vi "Write Frame (Binary).vi"(8 "error in (no error)":errorcluster, 9 "timeout (1000 ms)":i32=1000, 10 "Bytes":u8[](array[numeric]) format="%08b", 11 "Connection.WS":refnum<class "Connection.WS.lvclass">) -> (0 "error out":errorcluster, 3 "Connection.WS":refnum<class "Connection.WS.lvclass">)   [LabVIEW 2013, in "Connection.WS_GOSPL.lvlib" / "Connection.WS.lvclass"]
uses:
  Connection.WS.lvclass
  Websocket Frame Type -- ring.ctl
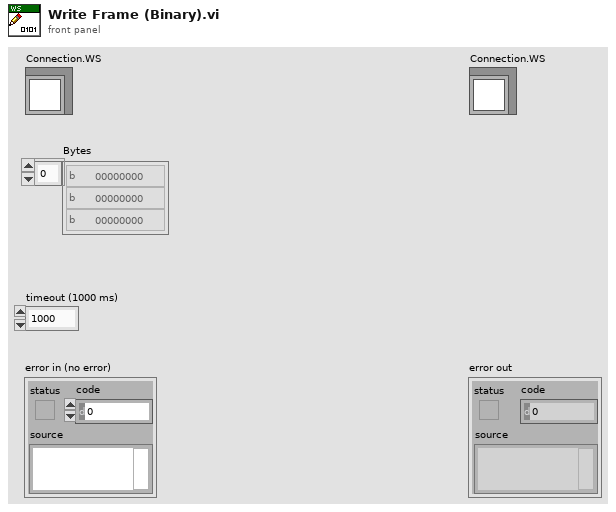
[diagram p1: front panel]
types:
  T1 = typedef "Connection.WS_GOSPL.lvlib/Connection.WS.lvclass/Websocket Frame Type -- ring.ctl" = u8
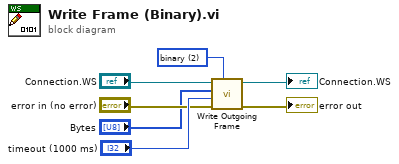
[diagram p0: block diagram]
diagram:
  w7 = T1 2 items=["continuation"=0, "text"=1, "binary"=2, "close"=8, "ping"=9, "pong"=10] ("x")
  n1 = call "Write Outgoing Frame.vi"("Frame type"=w7, "error in (no error)"="error in (no error)", "timeout ms (2000)"="timeout (1000 ms)", "Bytes"="Bytes", "Connection.WS"="Connection.WS") -> ("error out"=→"error out":errorcluster, "Connection.WS"=→"Connection.WS":refnum<class "Connection.WS.lvclass">)  [unwired: 5 in]
